vi "Create.vi"(4 "Buckets":dbl[](array[numeric])=[0.005, 0.01, 0.05, 0.1, 1.0, 10.0], 5 "OpenMetrics Compliant?":bool=TRUE, 6 "Label Names":string[](array[string]), 7 "Registry Name":string="_default_registry", 8 "error in (no error)":errorcluster, 9 "Auto-register?":bool=TRUE, 10 "Description":string, 11 "Name":string) -> (0 "error out":errorcluster, 3 "Histogram Ref":refnum<data-value>)   [LabVIEW 2020, in "Metrics.lvlib" / "Histogram.lvclass"]
doc: "Creates an histogram metric. An histogram uses threshold values that help categorizing how critical the metric value may get. An histogram metric which buckets are [0.1, 1, 10] and which value is observed to be 3 will increment the '0.1' and '1' buckets by one."
uses:
  Histogram.lvclass
  C:/Github-locals/PromVIEW/src/metrics/metric/Metric.lvclass
  metric/Metric.lvclass/Metric.ctl
  Histogram.lvclass/Histogram.ctl
  metric/Write Name.vi
  metric/Write Description.vi
  metric/Write Label Names.vi
  metric/Validate Name.vi
  registry/session/Registry Session.lvclass
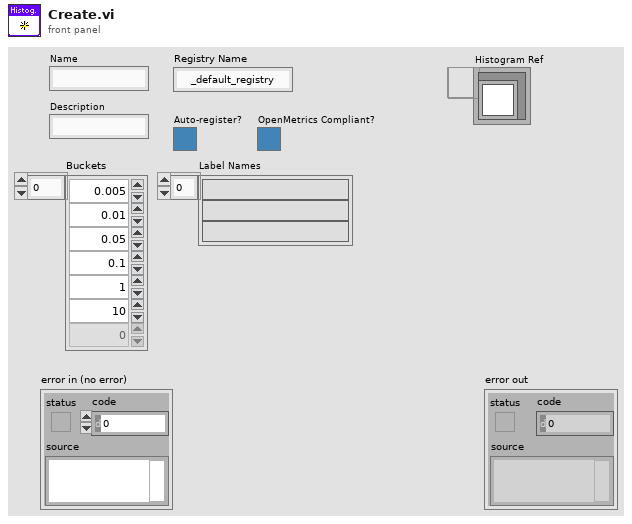
[diagram p1: front panel]
types:
  T1 = typedef "Registry.lvlib/Registry Session.lvclass/Session Handle.ctl" = refnum<data-value>
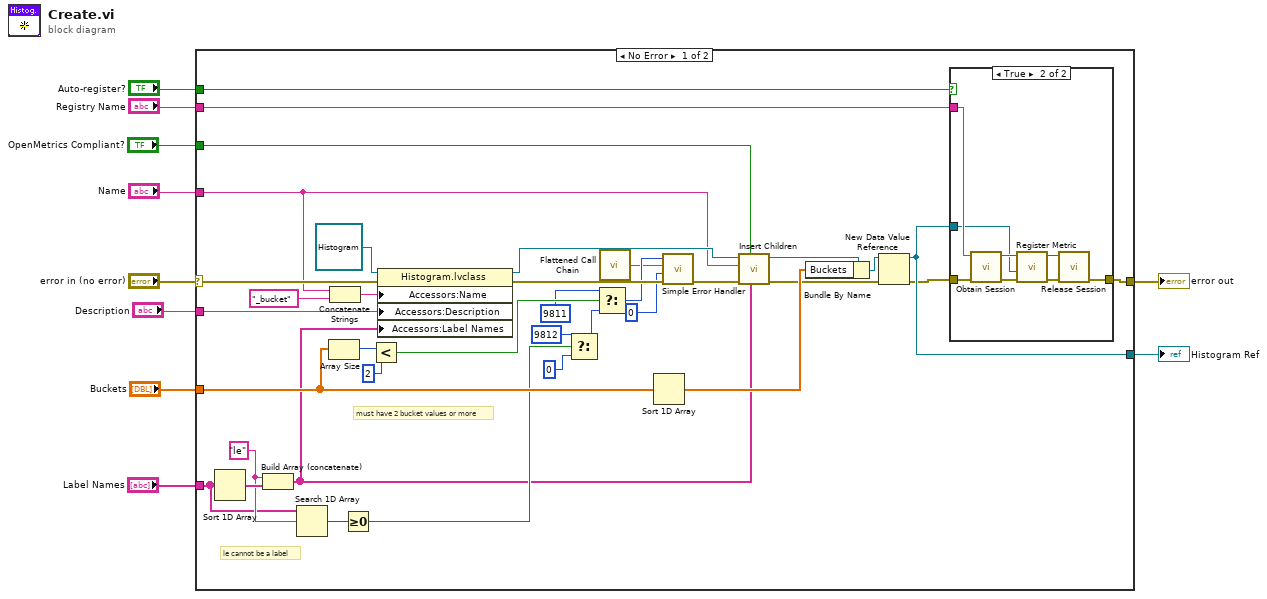
[diagram p0: block diagram]
diagram:
  n1 = case shown="No Error" "error in (no error)" {
    selector: "error in (no error)" -> [w33 w56]
    tunnel: [w40 w56] -> w9
    tunnel: "Description" -> [w46 _]
    tunnel: "Name" -> [w19 _]
    tunnel: "Label Names" -> [w14 _]
    tunnel: "Buckets" -> [w37 _]
    tunnel: "Auto-register?" -> [w44 _]
    tunnel: "Registry Name" -> [w43 _]
    tunnel: [w42 _] -> w3
    tunnel: "OpenMetrics Compliant?" -> [w23 _]
    frame No Error {
      w15 = "le" ("key")
      # "must have 2 bucket values or more"
      # "le cannot be a label"
      n2 = Sort 1D Array(array=w14) -> (sorted array=w16:string[])
      n3 = Build Array (concatenate)(w15, w16) -> (w13:string[])
      n4 = Search 1D Array(1D array=w14, element=w15) -> (index of element=w26:i32)  [unwired: 1 in]
      n5 = Array Size(array=w37) -> (size(s)=w36:i32)
      n6 = Concatenate Strings(w19, "_bucket" ("string")) -> (w18:string)
      n7 = Greater Or Equal To 0?(x=w26) -> (x >= 0?=w25:bool)
      n8 = Less?(x=w36, y=2) -> (x < y?=w34:bool)
      n9 = property class="Histogram.lvclass"(reference=refnum<class "Histogram.lvclass"> refnum, error in=w33, "Accessors:Name"=w18, "Accessors:Description"=w46, "Accessors:Label Names"=w13) -> (reference out=w24:refnum<class "Histogram.lvclass">, error out=w30:errorcluster)
      n10 = Select(t=9812 ("error code (no error:0)"), s=w25, f=0 ("error code (no error:0)")) -> (s? t:f=w28:i32)
      n11 = Select(t=9811 ("error code (no error:0)"), s=w34, f=w28) -> (s? t:f=w27:i32)
      n12 = call "Flattened Call Chain.vi"() -> ("Flattened Call Chain"=w12:string)  [unwired: 5 in]
      n13 = Sort 1D Array(array=w37) -> (sorted array=w38:dbl[])
      n14 = call <vilib>:"Simple Error Handler.vi"("error code (no error:0)"=w27, "error source (\" \")"=w12, "type of dialog (OK msg:1)"=0 ("error code (no error:0)"), "error in (no error)"=w30) -> ("error out"=w22:errorcluster)  [unwired: 1 in, 4 out]
      n15 = call "Insert Children.vi"("Label Names"=w13, "OpenMetrics Compliant?"=w23, "error in (no error)"=w22, "Metric Name"=w19, "Histogram in"=w24) -> ("error out"=w21:errorcluster, "Histogram out"=w17:refnum<class "Histogram.lvclass">)  [unwired: 5 in]
      n16 = Bundle By Name(cluster=w17, "Buckets"=w38) -> (w45:refnum<class "Histogram.lvclass">)
      n17 = New Data Value Reference(data value=w45, error in=w21) -> (data value reference=w42:refnum<data-value>, error out=w41:errorcluster)
      n18 = case shown="True" w44 {
        tunnel: w43 -> [_ w55]
        tunnel: [w47 w49] -> w40
        tunnel: w42 -> [_ w52]
        tunnel: w41 -> [w47 w51]
        frame False {
        }
        frame True {
          n19 = call "Obtain Session.vi"("error in (no error)"=w51, "Session  Name ()"=w55) -> ("error out"=w53:errorcluster, "Session Handle"=w54:T1)  [unwired: 8 in]
          n20 = call "Register Metric.vi"("error in (no error)"=w53, "New Metric"=w52, "Session Handle in"=w54) -> ("error out"=w50:errorcluster, "Session Handle out"=w48:T1)  [unwired: 7 in]
          n21 = call "Release Session.vi"("error in (no error)"=w50, "Session Handle"=w48) -> ("error out"=w49:errorcluster)  [unwired: 9 in]
        }
      }
    }
    frame Error {
    }
  }
  "error out" <- w9
  "Histogram Ref" <- w3
